vi "Generate Animation DVR.vi"(8 "Error In":errorcluster, 11 "Animation In":refnum<class "Animation.lvclass">) -> (0 "Error Out":errorcluster, 3 "Animation Out":refnum<class "Animation.lvclass">)   [LabVIEW 2021, in "Animation.lvclass"]
uses:
  Animation.lvclass
  Controls/Data.ctl
  Animation.lvclass/Animation.ctl
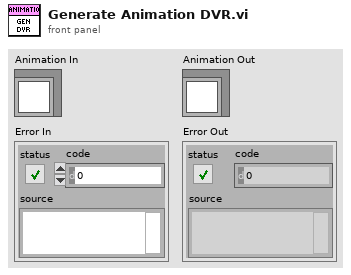
[diagram p1: front panel]
types:
  T1 = typedef "Animation.lvclass/Data.ctl" = cluster{"Tag":string}
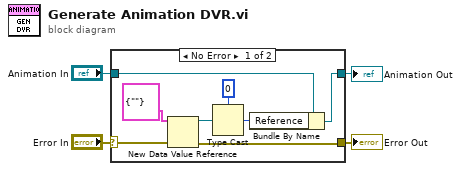
[diagram p0: block diagram]
diagram:
  n1 = case shown="No Error" "Error In" {
    selector: "Error In" -> [w12 w14]
    tunnel: "Animation In" -> [w9 w13]
    tunnel: [w6 w14] -> w1
    tunnel: [w7 w13] -> w3
    frame No Error {
      n2 = New Data Value Reference(data value=T1 {"Tag"=""} ("Data"), error in=w12) -> (data value reference=w10:refnum<data-value>, error out=w6:errorcluster)
      n3 = Type Cast(type=u64 0, x=w10) -> (*(type *) &x=w8:u64)
      n4 = Bundle By Name(cluster=w9, "Reference"=w8) -> (w7:refnum<class "Animation.lvclass">)
    }
    frame Error {
    }
  }
  "Animation Out" <- w3
  "Error Out" <- w1
